vi "Reset Interpreter.vi"(8 "error in (no error)":errorcluster, 11 "gScript Interpreter in":refnum<class "gScript Interpreter.lvclass">) -> (0 "error out":errorcluster, 3 "gScript Interpreter out":refnum<class "gScript Interpreter.lvclass">)   [LabVIEW 2017, in "gScript Interpreter.lvclass"]
uses:
  gScript Interpreter.lvclass
  gScript Interpreter.lvclass/gScript Interpreter.ctl
  Type Definitions/Error Mode.ctl
  Type Definitions/Label.ctl
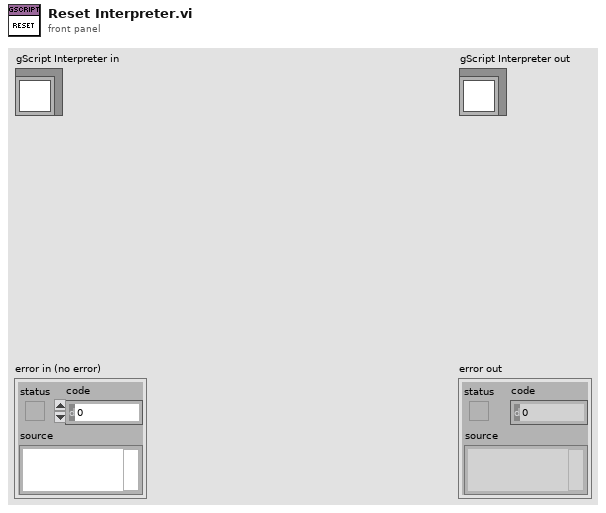
[diagram p1: front panel]
types:
  T1 = typedef "Label.ctl" = cluster{"Label":string, "Line":i32, "Arguments":string[]}
  T2 = typedef "Error Mode.ctl" = enum16{"default", "prompt", "setvar"}
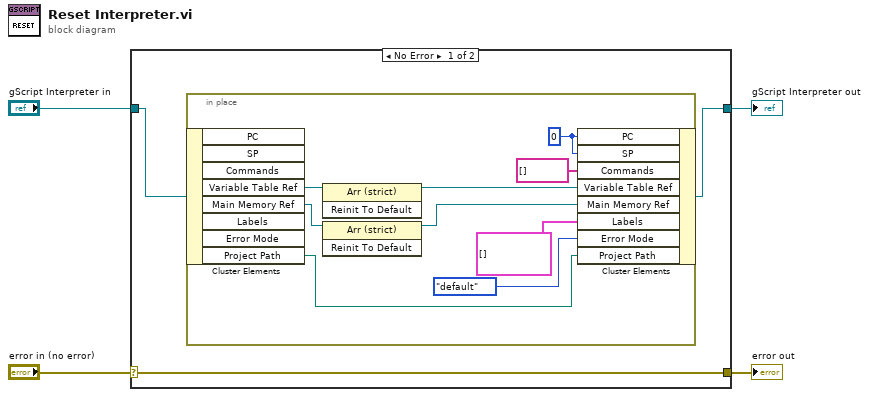
[diagram p0: block diagram]
diagram:
  n1 = case shown="No Error" "error in (no error)" {
    selector: "error in (no error)" -> [w5 w18]
    tunnel: [w5 w18] -> w3
    tunnel: [w6 w17] -> w1
    tunnel: "gScript Interpreter in" -> [w7 w17]
    frame No Error {
      n2 = in-place {
        w16 = 0 ("PC")
        n3 = in-place-cluster #1(w7) -> ("Variable Table Ref"=w14:refnum<vi>, "Main Memory Ref"=w11:refnum<vi>, "Project Path"=w8:path)  [unwired: 5 out]
        n4 = invoke class="Arr (strict)" method="Reinit To Default"(reference=w14) -> (reference out=w13:refnum<vi>)  [unwired: 2 in, 2 out]
        n5 = invoke class="Arr (strict)" method="Reinit To Default"(reference=w11) -> (reference out=w10:refnum<vi>)  [unwired: 2 in, 2 out]
        n6 = in-place-cluster #1("PC"=w16, "SP"=w16, "Commands"=string[] [], "Variable Table Ref"=w13, "Main Memory Ref"=w10, "Labels"=T1[] [], "Error Mode"=Error_Mode."default", "Project Path"=w8) -> (w6:refnum<class "gScript Interpreter.lvclass">)
      }
    }
    frame Error {
    }
  }
  "error out" <- w3
  "gScript Interpreter out" <- w1
